vi "Resolve Response Linkaging.vi"(7 "Response Refnum in":T2 format="%.0x", 8 "error in (no error)":errorcluster, 10 "Response Format":string, 11 "Linked Channels":T1[](array[typedef]) {"Channel Refnum" format="%.0x"}) -> (0 "error out":errorcluster, 2 "Linked Channels out":T3[](array[typedef]))   [LabVIEW 2018, in "Instrument Addon Scripting API.lvlib"]
uses:
  Instrument Addon Scripting API.lvlib
  Addon/Addon Shared/Types/Linked Channel Cluster.ctl
  <vilib>/NI Veristand/Custom Device API/Custom Device Item Ref.ctl
  TypeDefs/Linked Channel.ctl
  <vilib>/NI Veristand/Custom Device API/Custom Device API.lvlib
  Addon/Addon Shared/Instrument Addon Shared.lvlib
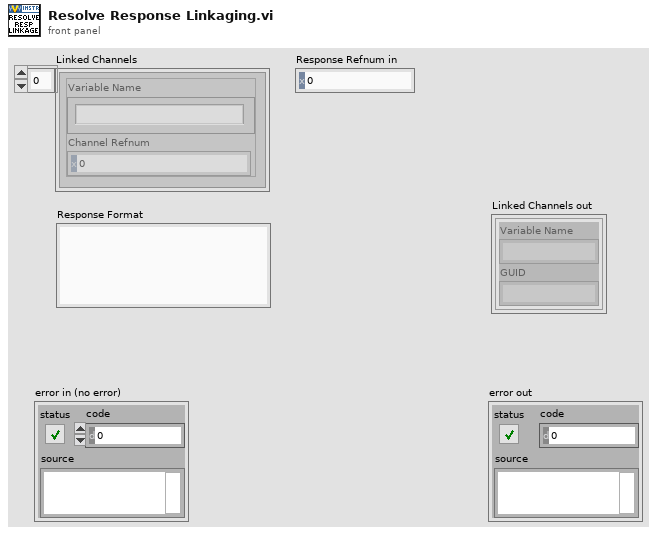
[diagram p1: front panel]
types:
  T1 = typedef "Instrument Addon Scripting API.lvlib/Linked Channel.ctl" = cluster{"Variable Name":string, "Channel Refnum":T2}
  T2 = typedef "Custom Device API.lvlib/Custom Device Item Ref.ctl" = u64
  T3 = typedef "Instrument Addon Shared.lvlib/Linked Channel Cluster.ctl" = cluster{"Variable Name":string, "GUID":string}
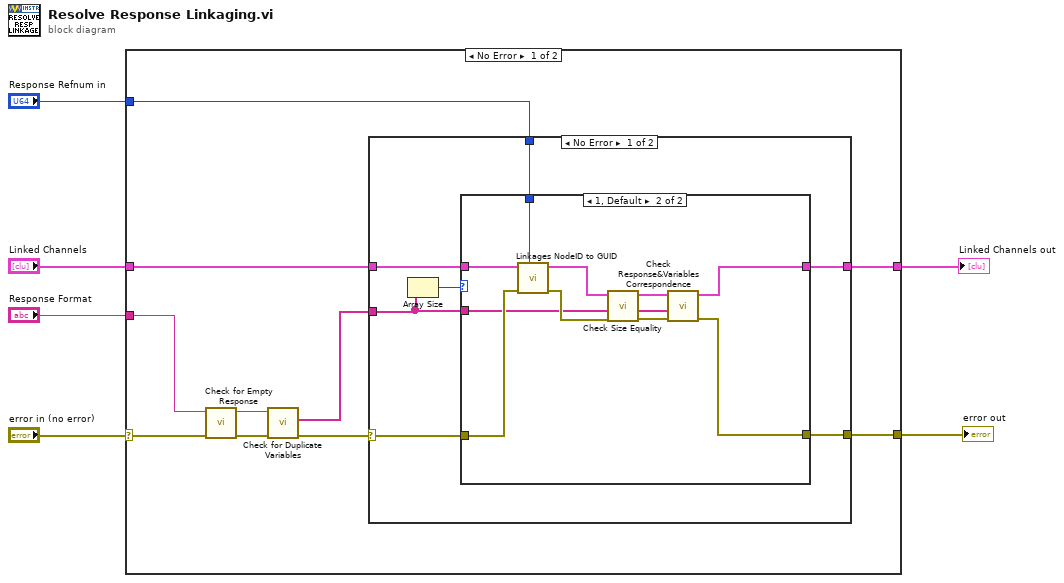
[diagram p0: block diagram]
diagram:
  n1 = case shown="No Error" "error in (no error)" {
    selector: "error in (no error)" -> [w12 w37]
    tunnel: [w16 w37] -> w6
    tunnel: [w15 _] -> w5
    tunnel: "Response Refnum in" -> [w14 _]
    tunnel: "Linked Channels" -> [w13 _]
    tunnel: "Response Format" -> [w10 _]
    frame No Error {
      n2 = call "Check for Empty Response.vi"("Error In"=w12, "Response Format in"=w10) -> ("Error Out"=w11:errorcluster, "Response Format out"=w9:string)  [unwired: 8 in]
      n3 = call "Check for Duplicate Variables.vi"("error in (no error)"=w11, "Response Format in"=w9) -> ("error out"=w8:errorcluster, "Variables"=w7:string[])  [unwired: 7 in, 1 out]
      n4 = case shown="No Error" w8 {
        selector: w8 -> [w18 w36]
        tunnel: [w23 w36] -> w16
        tunnel: w13 -> [w22 _]
        tunnel: w7 -> [w21 _]
        tunnel: [w20 _] -> w15
        tunnel: w14 -> [w19 _]
        frame No Error {
          n5 = Array Size(array=w21) -> (size(s)=w17:i32)
          n6 = case shown="1, Default" w17 {
            tunnel: w22 -> [_ w35]
            tunnel: w18 -> [w24 w34]
            tunnel: [w24 w31] -> w23
            tunnel: w21 -> [_ w30]
            tunnel: [_ w29] -> w20
            tunnel: w19 -> [_ w28]
            frame 0 {
            }
            frame 1, Default {
              n7 = call "Linkages NodeID to GUID.vi"("Response Refnum in"=w28, "error in (no error)"=w34, "Linked Channels in"=w35) -> ("error out"=w33:errorcluster, "Linked Channels out"=w32:cluster{"Variable Name":string, "GUID":string}[])  [unwired: 7 in]
              n8 = call "Check Size Equality.vi"("Error In"=w33, "Variables"=w30, "Linked Channels in"=w32) -> ("Error Out"=w27:errorcluster, "Variables out"=w25:string[], "Linked Channels out"=w26:cluster{"Variable Name":string, "GUID":string}[])  [unwired: 6 in]
              n9 = call "Check Response&Variables Correspondence.vi"("error in (no error)"=w27, "Variables in"=w25, "Linked Channels in"=w26) -> ("error out"=w31:errorcluster, "Linked Channels out"=w29:T3[])  [unwired: 7 in]
            }
          }
        }
        frame Error {
        }
      }
    }
    frame Error {
    }
  }
  "error out" <- w6
  "Linked Channels out" <- w5
